vi "Fgen Arb Tester.vi"() -> ()   [LabVIEW 2011]
doc: "This example shows how to use Script mode. This is a basic example that shows how to generate waveforms according to a script. Configuring a script trigger that is used as a start trigger is optional.\n\nThere are various options for the script to be used. Consult the Script control help for more information on configuring the example for specific scripts."
uses:
  <instrlib>/niFgen/niFgen.llb/niFgen_ctl Trigger Script - trigID Values (Ring).ctl
  <instrlib>/niFgen/niFgen.llb/niFgen Output Mode.ctl
  <instrlib>/niFgen/niFgen.llb/niFgen_ctl Exported Signal Identifiers (Ring).ctl
  <instrlib>/niFgen/niFgen.llb/niFgen_ctl Exported Signal Desination Values (ComboBox).ctl
  <instrlib>/niFgen/niFgen.llb/niFgen_ctl Exported Signal Name Values (Ring).ctl
  <instrlib>/niFgen/niFgen.llb/niFgen_ctl Trigger DigEdge - Edge Values (Ring).ctl
  <instrlib>/niFgen/niFgen.llb/niFgen_ctl Trigger DigLvl - Level Values (Ring).ctl
  <instrlib>/niFgen/niFgen.llb/niFgen_ctl Trigger SW - TrigName Values (Ring).ctl
  <instrlib>/niFgen/niFgen.llb/niFgen Disable Script Trigger.vi
  <instrlib>/niFgen/niFgen.llb/niFgen Configure Software Edge Script Trigger.vi
  <instrlib>/niFgen/niFgen.llb/niFgen Configure Digital Edge Script Trigger.vi
  <instrlib>/niFgen/niFgen.llb/niFgen Configure Digital Level Script Trigger.vi
  <instrlib>/niFgen/niFgen.llb/niFgen Write Named Waveform (I16).vi
panel:
  in  "Script Trigger Source":string(combo)="PFI0"
  in  "Script Trigger Type":u16(ring) items=["None", "Software Edge", "Digital Edge", "Digital Level"]
  in  "Trigger":bool caption="Send Software Trigger"
  in  "Scripts":string[](array[string])=["script myScript0\nrepeat forever\n    Generate wfmSine marker0(0)\nwait 2000\n  Generate wfmTriangle marker0(0)\nwait 2000\nend repeat\nend script", "script myScript1\n  Wait until scriptTrigger0\n  Generate wfmSquare\n  Generate wfmSine\n  Generate wfmTriangle\n  Generate wfmSine\n  Generate wfmDC0V\nend script", "script myScript2\n  Generate wfmSquare\n  Repeat 2\n    Generate wfmSine\n  end repeat\n  Repeat 5\n    Generate wfmTriangle\n  end repeat\n  Repeat 2\n    Generate wfmSine\n  end repeat\n  Repeat 3\n    Generate wfmDC0V\n  end repeat\nend script", "script myScript3\n  Wait until scriptTrigger0\n  Generate wfmSquare\n  Repeat 2\n    Generate wfmSine\n  end repeat\n  Repeat 5\n    Generate wfmTriangle\n  end repeat\n  Repeat 2\n    Generate wfmSine\n  end repeat\n  Repeat 3\n    Generate wfmDC0V\n  end repeat\nend script", "script myScript4\n  Repeat forever\n    Generate wfmSquare\n    Repeat 2\n      Generate wfmSine\n    end repeat\n    Repeat 5\n      Generate wfmTriangle\n    end repeat\n    Repeat 2\n      Generate wfmSine\n    end repeat\n    Repeat 3\n      Generate wfmDC0V\n    end repeat\n  end repeat\nend script", "script myScript5\n  Wait until scriptTrigger0\n  Repeat forever\n    Generate wfmSquare\n    Repeat 2\n      Generate wfmSine\n    end repeat\n    Repeat 5\n      Generate wfmTriangle\n    end repeat\n    Repeat 2\n      Generate wfmSine\n    end repeat\n    Repeat 3\n      Generate wfmDC0V\n    end repeat\n  end repeat\nend script"]
  in  "Waveform Information Array":T1(array[cluster])=[{"Name"="wfmSine", "Waveform"={"waveform type"=enum."sine", "amplitude"=1.0, "# of points"=250}}, {"Name"="wfmSquare", "Waveform"={"waveform type"=enum."square", "amplitude"=1.0, "# of points"=1200}}, {"Name"="wfmTriangle", "Waveform"={"waveform type"=enum."triangle", "amplitude"=1.0, "# of points"=250}}, {"Name"="wfmDC0V", "Waveform"={"waveform type"=enum."DC Value", "amplitude"=0.0, "# of points"=256}}] {"Waveform"."amplitude" min=0.0 max=1.0 format="%.2f"}
  in  "Resource Name":refnum<k15>="PXI2Slot13"
  in  "Stop":bool caption="stop"
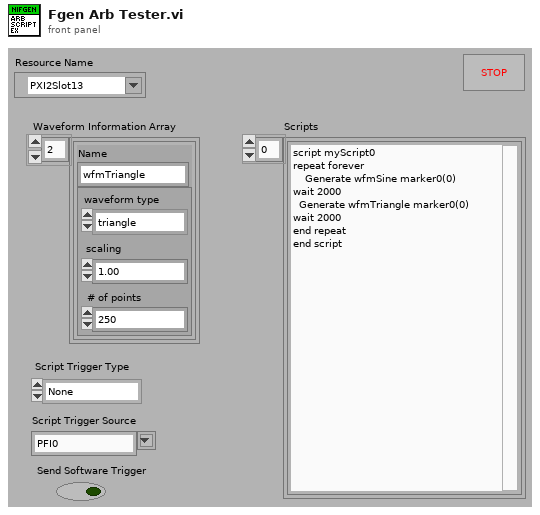
[diagram p1: front panel]
types:
  T1 = cluster{"Name":string, "Waveform":cluster{"waveform type":enum16{"sine", "cosine", "triangle", "square", "sawtooth", "increasing ramp", "decreasing ramp", "DC Value"}, "amplitude":dbl, "# of points":u32}}[]
  T2 = typedef "niFgen_ctl Exported Signal Name Values (Ring).ctl" = u16
  T3 = typedef "niFgen_ctl Exported Signal Desination Values (ComboBox).ctl" = string
  T4 = typedef "niFgen_ctl Exported Signal Identifiers (Ring).ctl" = string
  T5 = typedef "niFgen Output Mode.ctl" = u32
  T6 = typedef "niFgen_ctl Trigger Script - trigID Values (Ring).ctl" = string
  T7 = typedef "niFgen_ctl Trigger DigEdge - Edge Values (Ring).ctl" = i32
  T8 = typedef "niFgen_ctl Trigger DigLvl - Level Values (Ring).ctl" = i32
  T9 = cluster{"waveform type":enum16{"sine", "cosine", "triangle", "square", "sawtooth", "increasing ramp", "decreasing ramp", "DC Value"}, "amplitude":dbl, "# of points":u32}
  T10 = typedef "niFgen_ctl Trigger SW - TrigName Values (Ring).ctl" = i32
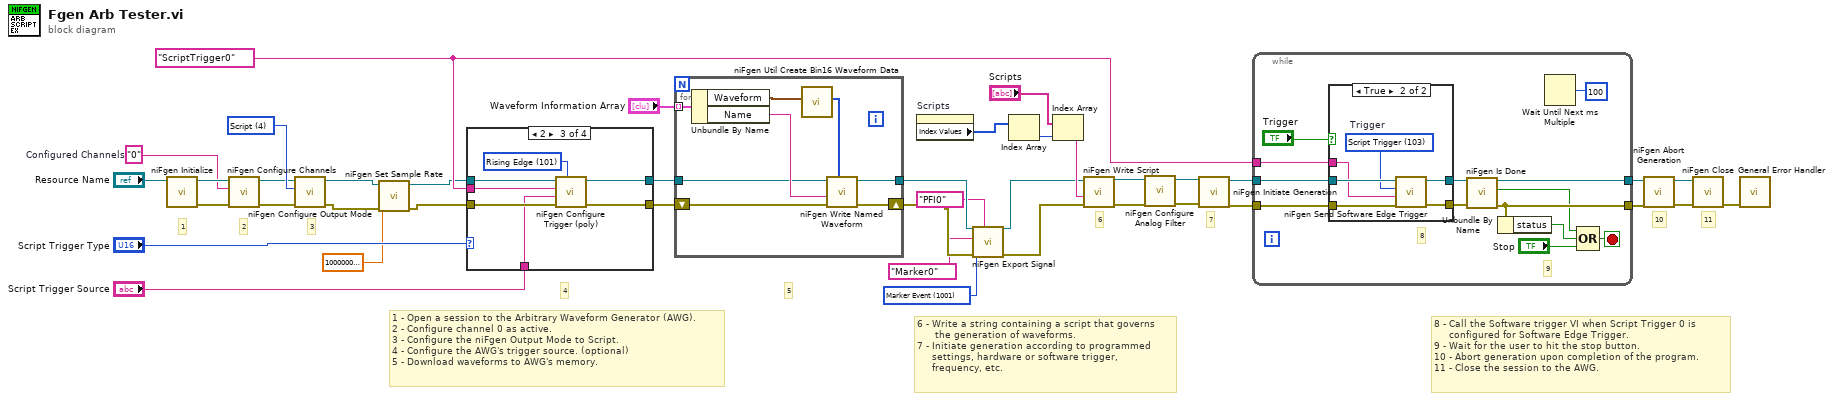
[diagram p0: block diagram]
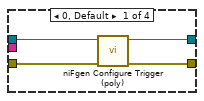
[diagram p2: hidden frame]
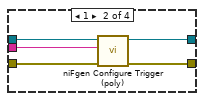
[diagram p3: hidden frame]
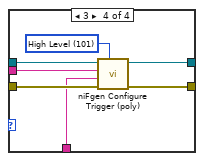
[diagram p4: hidden frame]
diagram:
  w10 = T2 1001 items=["Sample Clock"=101, "Sample Clock Timebase"=1006, "Reference Clock"=102, "Onboard Reference Clock"=1019, "Start Trigger"=1004, "Script Trigger"=103, "Marker Event"=1001, "Data Marker Event"=108, "Ready For Start Event"=105, "Started Event"=106, "Done Event"=107, "Synchronization Pulse"=1007, "Sync Out"=1002] ("Signal")
  w17 = "0"  # Configured Channels
  w22 = T5 4 items=["Standard Function", "Frequency List", "Arbitrary Waveform", "Arbitrary Sequence", "Script"] ("Output Mode")
  w23 = T6 "ScriptTrigger0" ("Trigger ID (Script Trigger 0)")
  # "2"
  # "6 - Write a string containing a script that governs \n      the generation of waveforms.\n7 - Initiate generation according to programmed \n     settings, hardware or software trigger, \n     frequency, etc."
  # "6"
  # "5"
  # "4"
  # "10"
  # "7"
  # "3"
  # "8 - Call the Software trigger VI when Script Trigger 0 is \n     configured for Software Edge Trigger.\n9 - Wait for the user to hit the stop button.\n10 - Abort generation upon completion of the program. \n11 - Close the session to the AWG."
  # "11"
  # "1"
  # "1 - Open a session to the Arbitrary Waveform Generator (AWG).\n2 - Configure channel 0 as active. \n3 - Configure the niFgen Output Mode to Script.\n4 - Configure the AWG's trigger source. (optional)\n5 - Download waveforms to AWG's memory."
  n1 = call <instrlib>:"niFgen Initialize.vi"("Resource Name"="Resource Name") -> ("error out"=w21:errorcluster, "Instrument Handle Out"=w18:refnum<k15>)  [unwired: 9 in]
  n2 = call <instrlib>:"niFgen Configure Channels.vi"("error in (no error)"=w21, "Channels"=w17, "Instrument Handle"=w18) -> ("error out"=w20:errorcluster, "Instrument Handle Out"=w19:refnum<k15>)  [unwired: 7 in]
  n3 = call <instrlib>:"niFgen Configure Output Mode.vi"("error in (no error)"=w20, "Output Mode (default: 0=Standard Function)"=w22, "Instrument Handle"=w19) -> ("error out"=w8:errorcluster, "Instrument Handle Out"=w9:refnum<k15>)  [unwired: 6 in]
  n4 = call <instrlib>:"niFgen Set Sample Rate.vi"("error in (no error)"=w8, "Sample Rate (Samp/s)"=100000000.0, "Instrument Handle"=w9) -> ("error out"=w7:errorcluster, "Instrument Handle Out"=w6:refnum<k15>)  [unwired: 7 in]
  n5 = case shown="2" "Script Trigger Type" {
    tunnel: w6 -> [w44 w49 w56 w63]
    tunnel: w7 -> [w43 w48 w55 w62]
    tunnel: [w42 w47 w54 w61] -> w27
    tunnel: [w41 w46 w53 w60] -> w26
    tunnel: "Script Trigger Source" -> [_ _ w52 w59]
    tunnel: w23 -> [_ w45 w51 w58]
    frame 0, Default {
      n6 = call-poly <instrlib>:"niFgen Configure Trigger (poly).vi"("error in (no error)"=w43, "Instrument Handle"=w44) -> ("error out"=w42:errorcluster, "Instrument Handle Out"=w41:refnum<k15>)  [unwired: 8 in]
    }
    frame 1 {
      n7 = call-poly <instrlib>:"niFgen Configure Trigger (poly).vi"("error in (no error)"=w48, "Trigger ID (Script Trigger 0)"=w45, "Instrument Handle"=w49) -> ("error out"=w47:errorcluster, "Instrument Handle Out"=w46:refnum<k15>)  [unwired: 7 in]
    }
    frame 2 {
      w50 = T7 101 items=["Rising Edge"=101, "Falling Edge"=102] ("Edge (Rising)")
      n8 = call-poly <instrlib>:"niFgen Configure Trigger (poly).vi"("Edge (Rising)"=w50, "error in (no error)"=w55, "Source"=w52, "Trigger ID (Script Trigger 0)"=w51, "Instrument Handle"=w56) -> ("error out"=w54:errorcluster, "Instrument Handle Out"=w53:refnum<k15>)  [unwired: 5 in]
    }
    frame 3 {
      w57 = T8 101 items=["High Level"=101, "Low Level"=102] ("Trigger When (High)")
      n9 = call-poly <instrlib>:"niFgen Configure Trigger (poly).vi"("Trigger When (High)"=w57, "error in (no error)"=w62, "Source"=w59, "Trigger ID (Script Trigger 0)"=w58, "Instrument Handle"=w63) -> ("error out"=w61:errorcluster, "Instrument Handle Out"=w60:refnum<k15>)  [unwired: 5 in]
    }
  }
  n10 = for {
    shift-right: [w67] -> w15
    shift-left: w27 -> [w65]
    tunnel: [w68] -> w13
    tunnel: w26 -> [w64]
    tunnel: "Waveform Information Array" -> [w71] mode=indexing
    n11 = Unbundle By Name(w71) -> ("Waveform"=w70:T9, "Name"=w66:string)
    n12 = call <instrlib>:"niFgen Util Create Bin16 Waveform Data.vi"("Waveform"=w70) -> ("Waveform Data"=w69:i16[])  [unwired: 10 in]
    n13 = call-poly <instrlib>:"niFgen Write Named Waveform.vi"("Waveform Data"=w69, "error in (no error)"=w65, "Waveform Name"=w66, "Instrument Handle"=w64) -> ("error out"=w67:errorcluster, "Instrument Handle Out"=w68:refnum<k15>)  [unwired: 5 in, 1 out]
  }
  n14 = property on="Scripts" class="Arr (strict)"() -> ("Index Values"=w30:u32[])  [unwired: 2 in, 2 out]
  n15 = call <instrlib>:"niFgen Export Signal.vi"("Output Terminal (do not export)"=T3 "PFI0", "error in (no error)"=w15, "Signal"=w10, "Signal Identifier (None)"=T4 "Marker0", "Instrument Handle"=w13) -> ("error out"=w14:errorcluster, "Instrument Handle Out"=w16:refnum<k15>)  [unwired: 5 in]
  n16 = Index Array(array=w30) -> (element=w29:u32)  [unwired: 1 in]
  n17 = Index Array(array="Scripts", index=w29) -> (element=w28:string)
  n18 = call <instrlib>:"niFgen Write Script.vi"("error in (no error)"=w14, "Script"=w28, "Instrument Handle"=w16) -> ("error out"=w3:errorcluster, "Instrument Handle Out"=w4:refnum<k15>)  [unwired: 7 in]
  n19 = call <instrlib>:"niFgen Configure Analog Filter.vi"("error in (no error)"=w3, "Instrument Handle"=w4) -> ("error out"=w2:errorcluster, "Instrument Handle Out"=w1:refnum<k15>)  [unwired: 8 in]
  n20 = call <instrlib>:"niFgen Initiate Generation.vi"("error in (no error)"=w2, "Instrument Handle"=w1) -> ("error out"=w37:errorcluster, "Instrument Handle Out"=w38:refnum<k15>)  [unwired: 8 in]
  n21 = while {
    tunnel: w37 -> [w82]
    tunnel: w38 -> [w83]
    tunnel: [w72] -> w35
    tunnel: [w74] -> w34
    tunnel: w23 -> [w81]
    stop <- w79 stop-if-true
    # "9"
    # "8"
    n22 = case shown="True" "Trigger" {
      tunnel: w83 -> [w86 w92]
      tunnel: w82 -> [w85 w91]
      tunnel: [w85 w90] -> w75
      tunnel: [w86 w89] -> w76
      tunnel: w81 -> [_ w87]
      frame False {
      }
      frame True {
        w88 = T10 103 items=["Start Trigger"=1004, "Script Trigger"=103]  # Trigger
        n23 = call <instrlib>:"niFgen Send Software Edge Trigger.vi"("error in (no error)"=w91, "Trigger ID (None)"=w87, "Trigger (Start Trigger)"=w88, "Instrument Handle"=w92) -> ("error out"=w90:errorcluster, "Instrument Handle Out"=w89:refnum<k15>)  [unwired: 6 in]
      }
    }
    n24 = call <instrlib>:"niFgen Is Done.vi"("error in (no error)"=w75, "Instrument Handle"=w76) -> ("error out"=w74:errorcluster, "Done"=w73:bool, "Instrument Handle Out"=w72:refnum<k15>)  [unwired: 7 in]
    n25 = Unbundle By Name(w74) -> ("status"=w77:bool)
    n26 = Wait Until Next ms Multiple(millisecond multiple=u32 100) -> ()  [unwired: 1 out]
    n27 = Compound Arithmetic op=OR(w73, w77, "Stop") -> (w79:bool)
  }
  n28 = call <instrlib>:"niFgen Abort Generation.vi"("error in (no error)"=w34, "Instrument Handle"=w35) -> ("error out"=w39:errorcluster, "Instrument Handle Out"=w40:refnum<k15>)  [unwired: 8 in]
  n29 = call <instrlib>:"niFgen Close.vi"("error in (no error)"=w39, "Instrument Handle"=w40) -> ("error out"=w32:errorcluster)  [unwired: 9 in]
  n30 = call <vilib>:"General Error Handler.vi"("error in (no error)"=w32) -> ()  [unwired: 10 in, 5 out]
